vi "Test Print Complex Numbers To Serial.vi"() -> ()   [LabVIEW 2014]
uses:
  <vilib>/Aledyne-TSXperts/Arduino Compatible Compiler for LabVIEW/Arduino Compatible Compiler for LabVIEW.lvlib
  <vilib>/Aledyne-TSXperts/Arduino Compatible Compiler for LabVIEW/addons/Complex Numbers/Complex Numbers.lvlib
panel:
  out "error out":errorcluster
  in  "error in (no error)":errorcluster
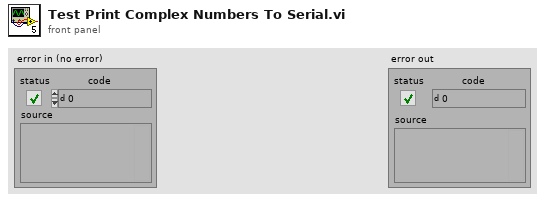
[diagram p1: front panel]
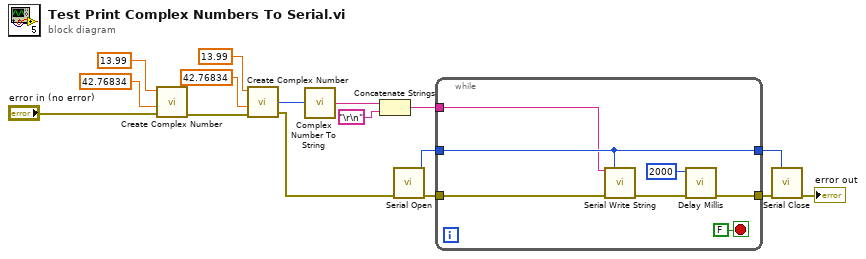
[diagram p0: block diagram]
diagram:
  n1 = call <vilib>:"Create Complex Number.vi"("Error In"="error in (no error)", "Imag"=42.76834, "Real"=13.99) -> ("Error Out"=w4:errorcluster)  [unwired: 2 in, 1 out]
  n2 = call <vilib>:"Create Complex Number.vi"("Error In"=w4, "Imag"=42.76834, "Real"=13.99) -> ("Error Out"=w2:errorcluster, "Complex"=w1:u32)  [unwired: 2 in]
  n3 = call <vilib>:"Complex Number To String.vi"("Complex number"=w1) -> ("String complex num."=w11:string)
  n4 = Concatenate Strings(w11, "\r\n") -> (w10:string)
  n5 = call <vilib>:"Serial Open.vi"("error in (no error)"=w2) -> ("Instance"=w14:u8, "error out"=w16:errorcluster)  [unwired: 13 in]
  n6 = while {
    tunnel: w16 -> [w22]
    tunnel: [w20] -> w15
    tunnel: w14 -> [w19]
    tunnel: [w19] -> w13
    tunnel: w10 -> [w18]
    stop <- FALSE stop-if-true
    n7 = call <vilib>:"Serial Write String.vi"("String"=w18, "Instance"=w19, "error in (no error)"=w22) -> ("error out"=w21:errorcluster)  [unwired: 12 in]
    n8 = call <vilib>:"Delay Millis.vi"("error in (no error)"=w21, "delay"=u32 2000) -> ("error out"=w20:errorcluster)  [unwired: 9 in]
  }
  n9 = call <vilib>:"Serial Close.vi"("Instance"=w13, "error in (no error)"=w15) -> ("error out"=→"error out":errorcluster)  [unwired: 13 in]
